vi "WriteToFile.vi"(8 "error in (no error)":errorcluster, 9 "Serialized JSON":string, 11 "ConverterBase in":refnum<class "FileConverterBase.lvclass">) -> (0 "error out":errorcluster, 3 "ConverterBase out":refnum<class "FileConverterBase.lvclass">)   [LabVIEW 2017, in "FileConverterBase.lvclass"]
uses:
  FileConverterBase.lvclass
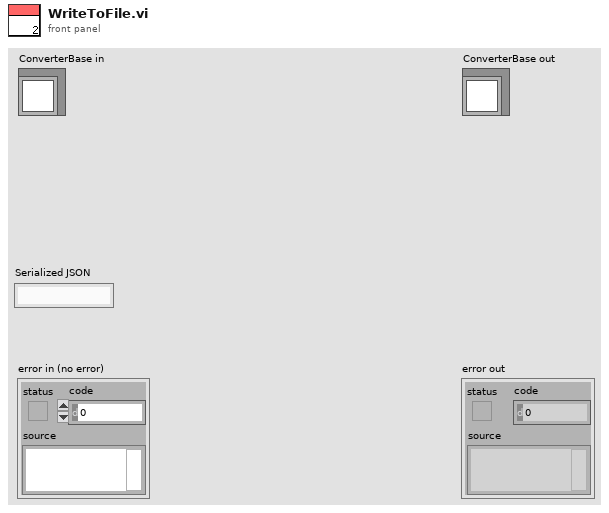
[diagram p1: front panel]
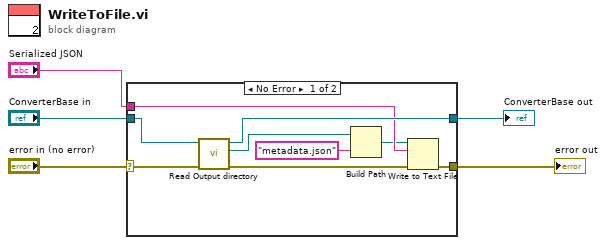
[diagram p0: block diagram]
diagram:
  n1 = case shown="No Error" "error in (no error)" {
    selector: "error in (no error)" -> [w12 w16]
    tunnel: [w14 w16] -> w4
    tunnel: [w10 w15] -> w2
    tunnel: "ConverterBase in" -> [w11 w15]
    tunnel: "Serialized JSON" -> [w9 _]
    frame No Error {
      n2 = call-dynamic "Read Output directory.vi"("error in (no error)"=w12, "FileConverterBase in"=w11) -> ("error out"=w13:errorcluster, "Output JSON File Path"=w8:path, "FileConverterBase out"=w10:refnum<class "FileConverterBase.lvclass">)  [unwired: 7 in]
      n3 = Build Path(base path=w8, name or relative path="metadata.json") -> (appended path=w6:path)
      n4 = Write to Text File(file (use dialog)=w6, text=w9, error in=w13) -> (error out=w14:errorcluster)  [unwired: 1 in, 2 out]
    }
    frame Error {
    }
  }
  "error out" <- w4
  "ConverterBase out" <- w2
